vi "4.vi"() -> ()   [LabVIEW 2015]
panel:
  out "Array":path[](array[path])
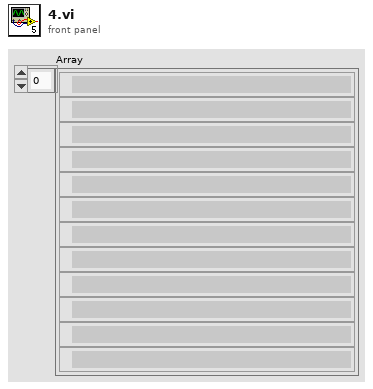
[diagram p1: front panel]
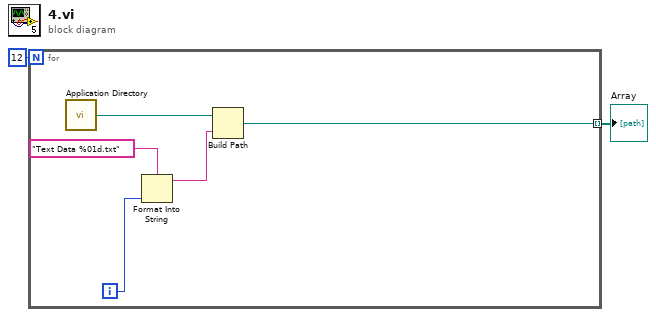
[diagram p0: block diagram]
diagram:
  n1 = for {
    N: 12 -> [_]
    tunnel: [w4] -> w1 mode=indexing
    i -> [w6]
    n2 = call <vilib>:"Application Directory.vi"() -> ("Application Directory"=w7:path)
    n3 = Format Into String(format string="Text Data %01d.txt", w6) -> (resulting string=w5:string)  [unwired: 2 in, 1 out]
    n4 = Build Path(base path=w7, name or relative path=w5) -> (appended path=w4:path)
  }
  "Array" <- w1
